vi "AlarmSetState.vi"(10 "Alarm State":string, 11 "Full Alarm Path":string) -> (0 "error out":errorcluster, 1 "Alarm State Text":string, 2 "Alarm Name":string)   [LabVIEW 2015, in "ni-veristand-steps-runtime-lib.lvlib"]
uses:
  ni-veristand-steps-runtime-lib.lvlib
  <vilib>/NI Veristand/Execution/Alarm/NI_VS Alarm ExecutionAPI.lvlib
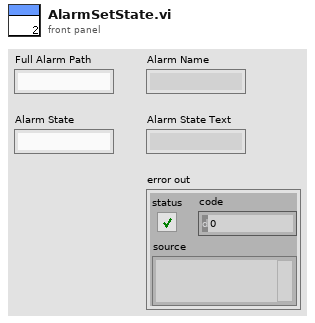
[diagram p1: front panel]
types:
  T1 = enum16{"Disabled", "Enabled", "Tripped", "Delayed Trip", "Indicate"}
  T2 = typedef "NI_VS Alarm ExecutionAPI.lvlib/AlarmAPI.ctl" = refnum<k24>
  T3 = typedef "NI_VS Alarm ExecutionAPI.lvlib/AlarmInfo.ctl" = cluster{"Watch Channel":string, "High Limit Constant":bool, "High Limit Channel":string, "High Limit":dbl, "Low Limit Constant":bool, "Low Limit Channel":string, "Low Limit":dbl, "Procedure Name":string, "Delay":dbl, "Trip Value":dbl, "Priority":enum16{"Low", "Medium", "High"}, "State":enum16{"Disabled", "Enabled", "Tripped", "Delayed Trip", "Indicate"}, "Mode":enum16{"Normal", "Indicate Only"}, "Group Number":u32, "Priority Number":u32, "Name":string, "Full Name":string}
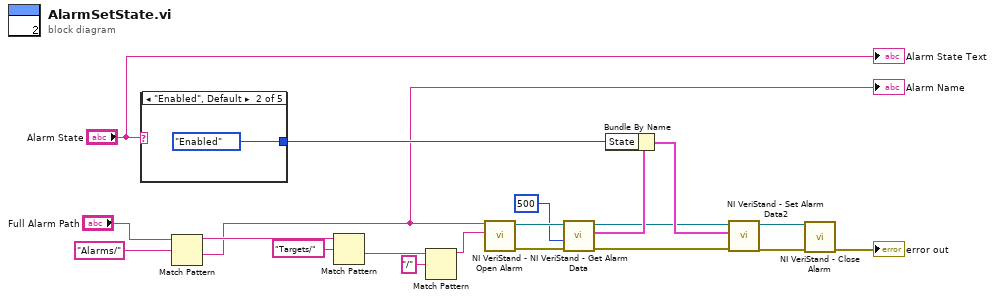
[diagram p0: block diagram]
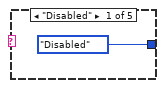
[diagram p2: hidden frame]
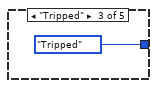
[diagram p3: hidden frame]
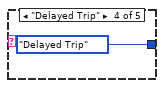
[diagram p4: hidden frame]
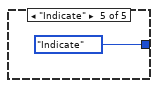
[diagram p5: hidden frame]
diagram:
  n1 = case shown="\"Enabled\", Default" "Alarm State" {
    tunnel: [T1."Disabled" ("State") T1."Enabled" ("State") T1."Tripped" ("State") T1."Delayed Trip" ("State") T1."Indicate" ("State")] -> w8
    frame "Disabled" {
    }
    frame "Enabled", Default {
    }
    frame "Tripped" {
    }
    frame "Delayed Trip" {
    }
    frame "Indicate" {
    }
  }
  n2 = Match Pattern(string="Full Alarm Path", regular expression="Alarms/") -> (before substring=w17:string, after substring=w2:string)  [unwired: 1 in, 2 out]
  "Alarm Name" <- w2
  n3 = Match Pattern(string=w17, regular expression="Targets/") -> (after substring=w20:string)  [unwired: 1 in, 3 out]
  n4 = Match Pattern(string=w20, regular expression="/") -> (before substring=w14:string)  [unwired: 1 in, 3 out]
  n5 = call <vilib>:"NI VeriStand - Open Alarm.vi"("Target Name (\"\": default target)"=w14, "Alarm Name"=w2) -> ("error out"=w12:errorcluster, "Alarm"=w13:T2)  [unwired: 8 in]
  n6 = call <vilib>:"NI VeriStand - Get Alarm Data.vi"("error in (no error)"=w12, "timeout (ms)"=u32 500, "Alarm in"=w13) -> ("error out"=w10:errorcluster, "Alarm Data"=w9:T3, "Alarm out"=w6:T2)  [unwired: 6 in]
  n7 = Bundle By Name(cluster=w9, "State"=w8) -> (w7:T3)
  n8 = call <vilib>:"NI VeriStand - Set Alarm Data2.vi"("error in (no error)"=w10, "Alarm Data"=w7, "Alarm in"=w6) -> ("error out"=w5:errorcluster, "Alarm out"=w4:T2)  [unwired: 7 in]
  n9 = call <vilib>:"NI VeriStand - Close Alarm.vi"("error in (no error)"=w5, "Alarm"=w4) -> ("error out"=→"error out":errorcluster)  [unwired: 9 in]
  "Alarm State Text" <- "Alarm State"
